vi "GT Compare Continue Pulse Mode.vi"(7 "standTime":i16, 8 "error in (no error)":errorcluster caption="错误输入（无错误）", 9 "count":i16, 10 "mode":i16, 11 "cardNum":i16) -> (0 "error out":errorcluster caption="错误输出", 3 "function return":i16)   [LabVIEW 2020, in "gts.lvlib"]
doc: "GT_API GT_CompareContinuePulseMode(short cardNum,short mode,short count,short standTime);"
uses:
  gts.lvlib
  dll/32bit/multi_card/gts.dll
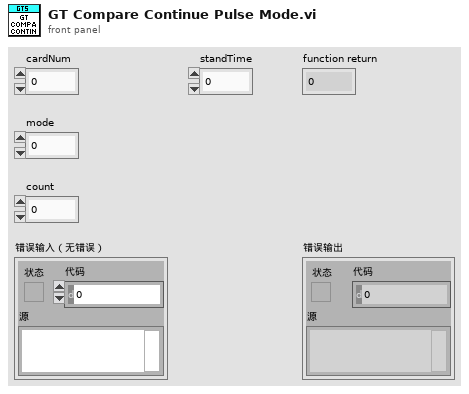
[diagram p1: front panel]
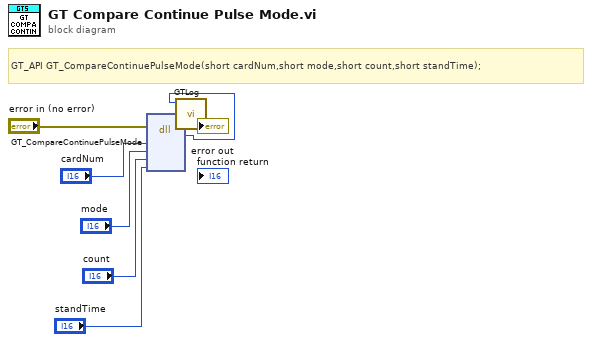
[diagram p0: block diagram]
diagram:
  # "GT_API GT_CompareContinuePulseMode(short cardNum,short mode,short count,short standTime);"
  n1 = dll-call lib="C:/1228/dll/32bit/multi_card/gts.dll" fn="GT_CompareContinuePulseMode"(error in="error in (no error)", "cardNum"="cardNum", "mode"="mode", "count"="count", "standTime"="standTime") -> (error out=w3:errorcluster, w1:i16)  [unwired: 6 in, 1 out]
  n2 = call "GTLog.vi"("error in (no error)"=w3, "Numeric"=w1) -> ("error out"=→"error out":errorcluster)  [unwired: 9 in]
